vi "DAQRead.vi"(0 "task/channels in":refnum<k21>, 9 "timeout":dbl=10.0 format="%0.2f", 11 "error in":errorcluster) -> (4 "task out":refnum<k21>, 6 "data":dbl[](array[numeric]) format="%0.2f", 15 "error out":errorcluster)   [LabVIEW 2010, in "PXIe-433x Custom Device.lvlib"]
doc: "Reads a single floating-point sample from each channel in a task that contains one or more analog input channels."
uses:
  PXIe-433x Custom Device.lvlib
  nilvaiu.dll
panel:
  # "channel"
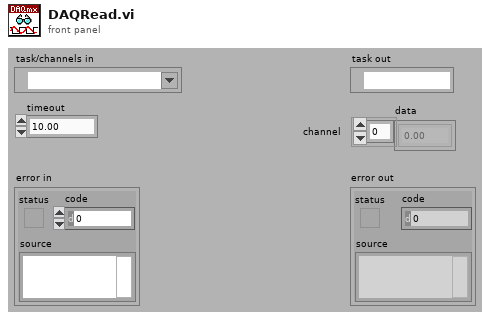
[diagram p1: front panel]
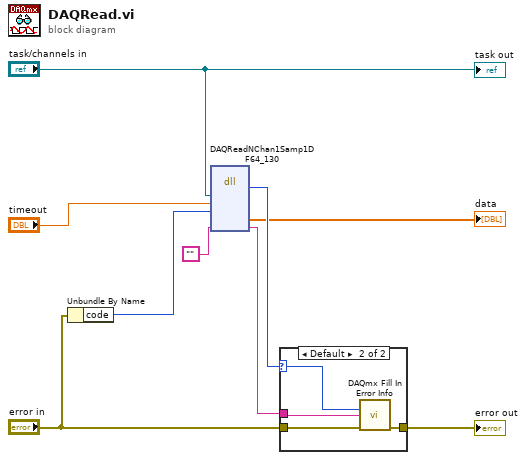
[diagram p0: block diagram]
diagram:
  n1 = Unbundle By Name("error in") -> ("code"=w2:i32)
  n2 = dll-call lib="nilvaiu.dll" fn="DAQReadNChan1Samp1DF64_130"("taskID"="task/channels in", "timeout"="timeout", "incomingStatus"=w2, "extendedErrorInfo"="") -> (w7:i32, "data"=→"data":dbl[], "extendedErrorInfo"=w5:string)  [unwired: 7 in, 2 out]
  n3 = case shown="Default" w7 {
    selector: w7 -> [_ w12]
    tunnel: "error in" -> [w10 w14]
    tunnel: [w10 w13] -> w9
    tunnel: w5 -> [_ w11]
    frame 0 {
    }
    frame Default {
      n4 = call <vilib>:"DAQmx Fill In Error Info.vi"("status code"=w12, "extended error info"=w11, "error in"=w14) -> ("error out"=w13:errorcluster)  [unwired: 12 in]
    }
  }
  "error out" <- w9
  "task out" <- "task/channels in"
